vi "Image_Get 32x32 Image Data.vi"(1 "new picture":picture) -> (0 "image data":T1)   [LabVIEW 2021]
uses:
  <vilib>/picture/picture.llb/imagedata.ctl
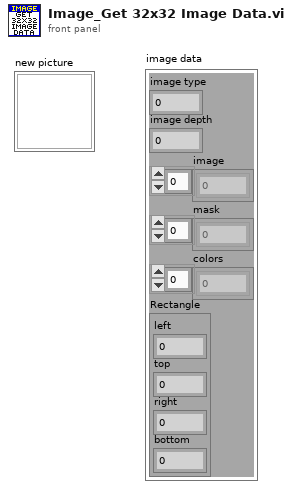
[diagram p1: front panel]
types:
  T1 = typedef "imagedata.ctl" = cluster{"image type":i32, "image depth":i32, "image":u8[], "mask":u8[], "colors":u32[], "Rectangle":cluster{"left":i16, "top":i16, "right":i16, "bottom":i16}}
  T2 = cluster{"left":i16, "top":i16, "right":i16, "bottom":i16}
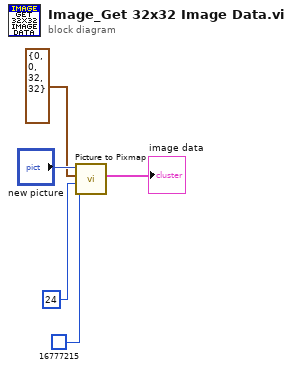
[diagram p0: block diagram]
diagram:
  n1 = call <vilib>:"Picture to Pixmap.vi"("Background Color"=u32 16777215, "depth"=24, "rect"=T2 {"left"=0, "top"=0, "right"=32, "bottom"=32}, "picture"="new picture") -> ("image data"=→"image data":T1)  [unwired: 7 out]
